vi "Project Springboard.vi"() -> ()   [LabVIEW 2015]
panel:
  out "Array":string[](array[string])
  out "Selected Item":string
  out "Current Name":string
  in  "COPY":bool
  in  "stop":bool
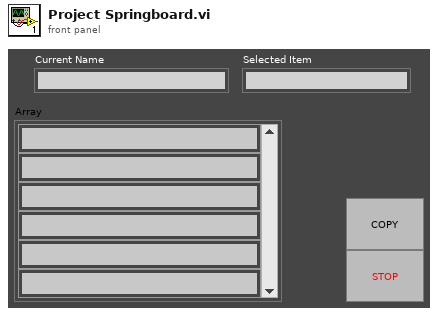
[diagram p1: front panel]
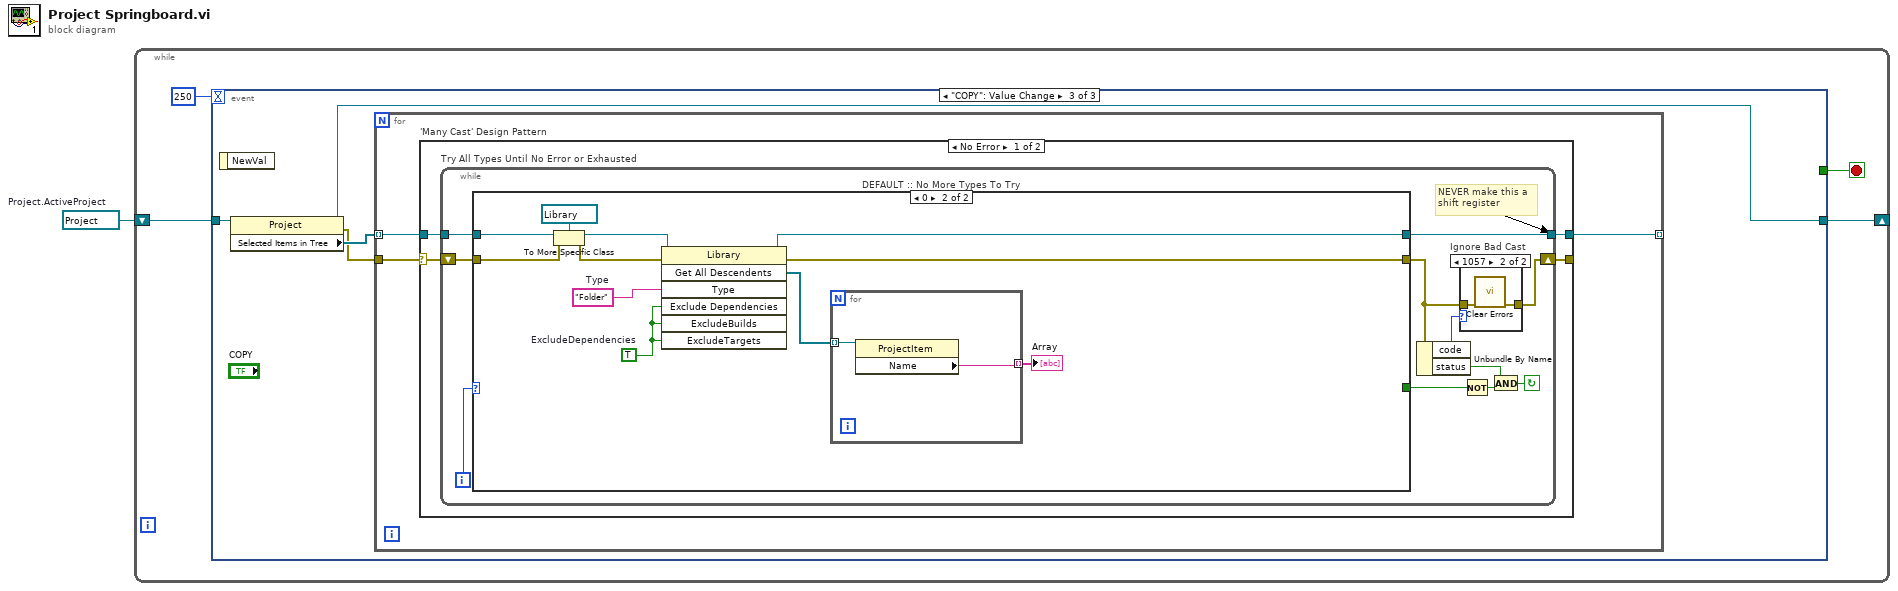
[diagram p0: block diagram]
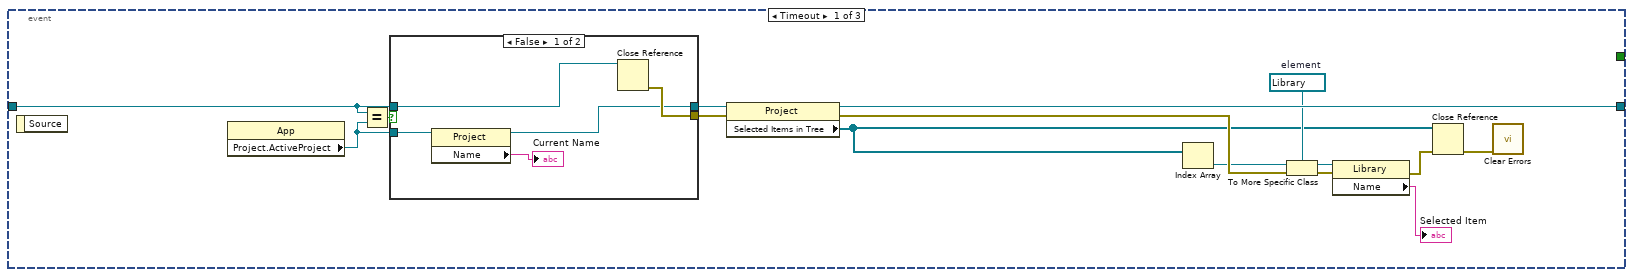
[diagram p2: hidden frame]
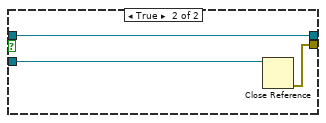
[diagram p3: hidden frame]
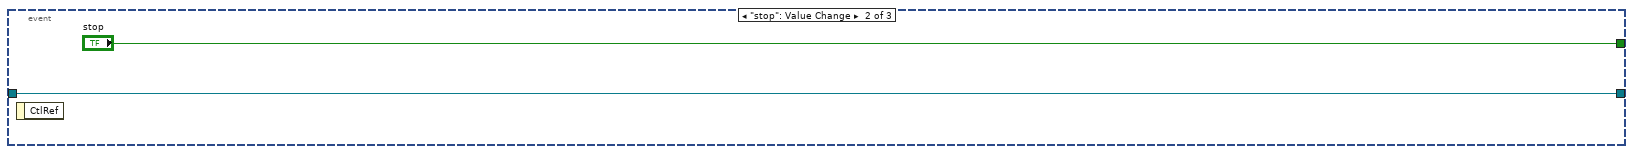
[diagram p4: hidden frame]
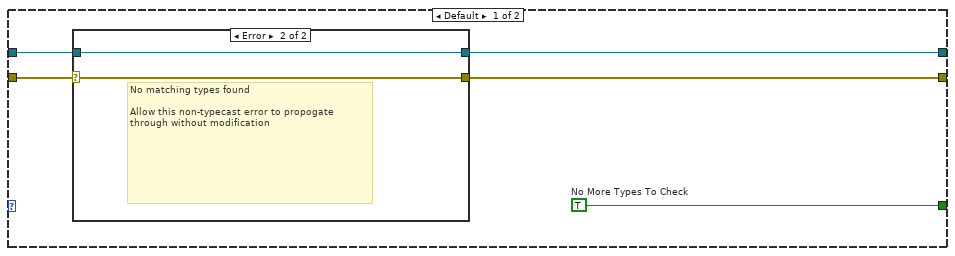
[diagram p6: hidden frame]
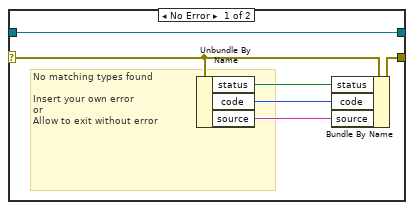
[diagram p7: hidden frame]
diagram:
  w1 = refnum<vi> refnum  # Project.ActiveProject
  n1 = while {
    shift-right: [w5] -> _
    shift-left: w1 -> [w4]
    stop <- w3 stop-if-true
    n2 = event shown="[2] \"COPY\": Value Change" {
      selector: _ -> [_ _ _]
      dyn-events: _ -> [_ _ _]
      timeout: 250 -> [_ _ _]
      tunnel: [w14 w30 w31] -> w5
      tunnel: w4 -> [w17 w30 w34]
      tunnel: [_ "stop" _] -> w3
      event Timeout {
        w8 = refnum<vi> refnum  # element
        n3 = event-data() -> ()  [unwired: 1 in, 1 out]
        n4 = property class="App"() -> ("Project.ActiveProject"=w18:refnum<vi>)  [unwired: 2 in, 2 out]
        n5 = Equal?(x=w17, y=w18) -> (x = y?=w19:bool)
        n6 = case shown="False" w19 {
          tunnel: w18 -> [w23 w28]
          tunnel: w17 -> [w25 w27]
          tunnel: [w22 w27] -> w15
          tunnel: [w24 w26] -> w11
          frame False {
            n7 = property class="Project"(reference=w23) -> (reference out=w22:refnum<vi>, "Name"=→"Current Name":string)  [unwired: 1 in, 1 out]
            n8 = Close Reference(reference=w25) -> (error out=w24:errorcluster)  [unwired: 1 in]
          }
          frame True {
            n9 = Close Reference(reference=w28) -> (error out=w26:errorcluster)  [unwired: 1 in]
          }
        }
        n10 = property class="Project"(reference=w15, error in=w11) -> (reference out=w14:refnum<vi>, error out=w20:errorcluster, "Selected Items in Tree"=w7:refnum<vi>[])
        n11 = Index Array(array=w7) -> (element=w13:refnum<vi>)  [unwired: 1 in]
        n12 = To More Specific Class(target class=w8, reference=w13, error in=w20) -> (specific class reference=w12:refnum<vi>, error out=w10:errorcluster)
        n13 = property class="Library"(reference=w12, error in=w10) -> (error out=w16:errorcluster, "Name"=→"Selected Item":string)  [unwired: 1 out]
        n14 = Close Reference(reference=w7, error in (no error)=w16) -> (error out=w9:errorcluster)
        n15 = call <vilib>:"Clear Errors.vi"("error in (no error)"=w9) -> ()  [unwired: 5 in, 2 out]
      }
      event "stop": Value Change {
        n16 = event-data() -> ()  [unwired: 1 in, 1 out]
      }
      event "COPY": Value Change {
        n17 = event-data() -> ()  [unwired: 1 in, 1 out]
        n18 = property class="Project"(reference=w34) -> (reference out=w31:refnum<vi>, error out=w32:errorcluster, "Selected Items in Tree"=w33:refnum<vi>[])  [unwired: 1 in]
        n19 = for {
          tunnel: w33 -> [w37] mode=indexing
          tunnel: w32 -> [w36]
          tunnel: [w35] -> _ mode=indexing
          n20 = case "'Many Cast' Design Pattern" shown="No Error" w36 {
            selector: w36 -> [w38 w83]
            tunnel: w37 -> [w41 w82]
            tunnel: [w40 w82] -> w35
            tunnel: [w39 w83] -> _
            frame No Error {
              n21 = while "Try All Types Until No Error or Exhausted" {
                tunnel: w41 -> [w52]
                tunnel: [w51] -> w40
                shift-right: [w44] -> w39
                shift-left: w38 -> [w46]
                i -> [w50]
                stop <- w49 continue-if-true
                # "NEVER make this a\nshift register"
                n22 = case "DEFAULT :: No More Types To Try" shown="0" w50 {
                  tunnel: w46 -> [w57 w79]
                  tunnel: w52 -> [w58 w77]
                  tunnel: [w59 w74] -> w51
                  tunnel: [w56 w73] -> w43
                  tunnel: [w60 _] -> w48
                  frame Default {
                    w60 = TRUE  # No More Types To Check
                    n23 = case shown="Error" w57 {
                      selector: w57 -> [w64 w67]
                      tunnel: [w66 w68] -> w59
                      tunnel: w58 -> [w66 w68]
                      tunnel: [w65 w67] -> w56
                      frame No Error {
                        # "No matching types found\n\nInsert your own error \nor\nAllow to exit without error"
                        n24 = Unbundle By Name(w64) -> ("status"=w63:bool, "code"=w62:i32, "source"=w61:string)
                        n25 = Bundle By Name(cluster=w64, "status"=w63, "code"=w62, "source"=w61) -> (w65:errorcluster)
                      }
                      frame Error {
                        # "No matching types found\n\nAllow this non-typecast error to propogate through without modification"
                      }
                    }
                  }
                  frame 0 {
                    w69 = "Folder"  # Type
                    w72 = TRUE  # ExcludeDependencies
                    n26 = To More Specific Class(target class=refnum<vi> refnum ("Waveform Chart"), reference=w77, error in=w79) -> (specific class reference=w75:refnum<vi>, error out=w76:errorcluster)
                    n27 = invoke class="Library" method="Get All Descendents"(reference=w75, error in=w76, "Type"=w69, "Exclude Dependencies"=w72, "ExcludeBuilds"=w72, "ExcludeTargets"=w72) -> (reference out=w74:refnum<vi>, error out=w73:errorcluster, "All Descendents"=w71:refnum<vi>[])  [unwired: 1 in, 4 out]
                    n28 = for {
                      tunnel: w71 -> [w81] mode=indexing
                      tunnel: [w80] -> w70 mode=indexing
                      n29 = property class="ProjectItem"(reference=w81) -> ("Name"=w80:string)  [unwired: 1 in, 2 out]
                    }
                    "Array" <- w70
                  }
                }
                n30 = Unbundle By Name(w43) -> ("code"=w42:i32, "status"=w45:bool)
                n31 = case "Ignore Bad Cast" shown="1057" w42 {
                  tunnel: [w53 w55] -> w44
                  tunnel: w43 -> [w53 w54]
                  frame Default {
                  }
                  frame 1057 {
                    n32 = call <vilib>:"Clear Errors.vi"("error in (no error)"=w54) -> ("error out"=w55:errorcluster)  [unwired: 5 in, 1 out]
                  }
                }
                n33 = Not(x=w48) -> (.not. x?=w47:bool)
                n34 = And(x=w45, y=w47) -> (x .and. y?=w49:bool)
              }
            }
            frame Error {
            }
          }
        }
      }
    }
  }
